vi "Show Nested Panel.vi"(8 "error in":errorcluster, 10 "Panel Ident":string, 11 "Series Actor in":refnum<class "Series Actor.lvclass">) -> (0 "error out":errorcluster, 3 "Series Actor out":refnum<class "Series Actor.lvclass">)   [LabVIEW 2024, in "Series Actor.lvlib" / "Series Actor.lvclass"]
uses:
  Series Actor.lvclass
  <vilib>/ActorFramework/Message Enqueuer/Message Enqueuer.lvclass
  Series Actor.lvclass/Series Actor.ctl
  <vilib>/MGI/Panel Manager/Panel Actor/Panel Actor Messages/Show Panel Msg/Show Panel Msg.lvclass
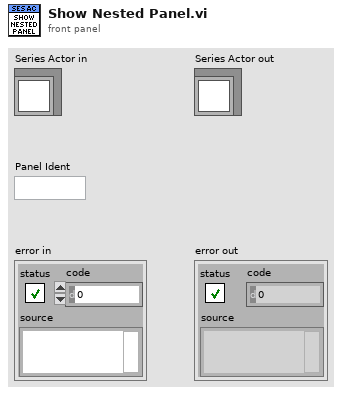
[diagram p1: front panel]
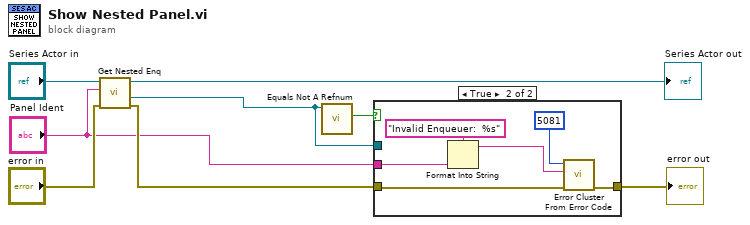
[diagram p0: block diagram]
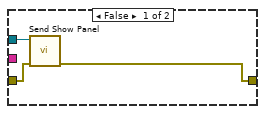
[diagram p2: hidden frame]
diagram:
  n1 = call "Get Nested Enq.vi"("error in"="error in", "Ident"="Panel Ident", "Series Actor in"="Series Actor in") -> ("error out"=w2:errorcluster, "Enq"=w3:refnum<class "Message Enqueuer.lvclass">, "Series Actor out"=→"Series Actor out":refnum<class "Series Actor.lvclass">)  [unwired: 6 in]
  n2 = call <vilib>:"Equals Not A Refnum.vi"("Message Enqueuer"=w3) -> ("Not a refnum?"=w7:bool)  [unwired: 10 in]
  n3 = case shown="True" w7 {
    tunnel: w3 -> [w11 _]
    tunnel: w2 -> [w10 w16]
    tunnel: [w9 w17] -> w8
    tunnel: "Panel Ident" -> [_ w13]
    frame False {
      n4 = call <vilib>:"Send Show Panel.vi"("Error In"=w10, "Message Enqueuer in"=w11) -> ("Error Out"=w9:errorcluster)  [unwired: 8 in, 1 out]
    }
    frame True {
      n5 = Format Into String(format string="Invalid Enqueuer:  %s" ("error message (\"\")"), w13) -> (resulting string=w12:string)  [unwired: 2 in, 1 out]
      n6 = call <vilib>:"Error Cluster From Error Code.vi"("error in (no error)"=w16, "error message (\"\")"=w12, "error code (0)"=5081) -> ("error out"=w17:errorcluster)  [unwired: 6 in]
    }
  }
  "error out" <- w8
